vi "BBB Blink.vi"() -> ()   [LabVIEW 2025]
doc: "Automatically blink and LED attached to a digital output channel of a LINX device."
uses:
  <vilib>/MakerHub/LINX/Public/Peripherals/Digital/Digital Write N Chans.vi
  <vilib>/MakerHub/LINX/Public/Peripherals/Digital/Digital Read N Chans.vi
  <vilib>/MakerHub/LINX/Private/Local IO/LinxDigitalWrite.vi
  <vilib>/MakerHub/LINX/Public/Utilities/Check Channel.vi
  <vilib>/MakerHub/LINX/Private/Local IO/LinxDigitalRead.vi
  <vilib>/MakerHub/LINX/Private/Local IO/Handle Errors.vi
  <vilib>/MakerHub/LINX/Private/Utilties/Generate Error.vi
  <vilib>/MakerHub/LINX/Public/Peripherals/PWM/PWM Set Duty Cycle N Chans.vi
  <vilib>/MakerHub/LINX/Public/Peripherals/Digital/Digital Write 1 Chan.vi
  <vilib>/MakerHub/LINX/Public/Peripherals/Digital/Digital Read 1 Chan.vi
  <vilib>/MakerHub/LINX/Public/Utilities/Open Local.vi
  <vilib>/MakerHub/LINX/LMH-LINX.lvlib
panel:
  out "DI Value":bool
  in  "Digital Input Channel":u8=8
  out "DO Value":bool
  in  "Digital Output Channel":u8=7
  out "Loop Rate (Hz)":u32=4
  in  "Stop Button":bool
  # "LINX Device Settings"
  # "LED Value"
  # "Blink (Serial Interface)\n\nThis example demonstrates how to blink an LED on a LINX device connected to \nthe host computer using USB / Serial.\n\nInstructions\n1. Select the Serial Port associated with the LINX Device.\n2. Select the Digital Pin connected to the LED.\n3. Click the Run Arrow."
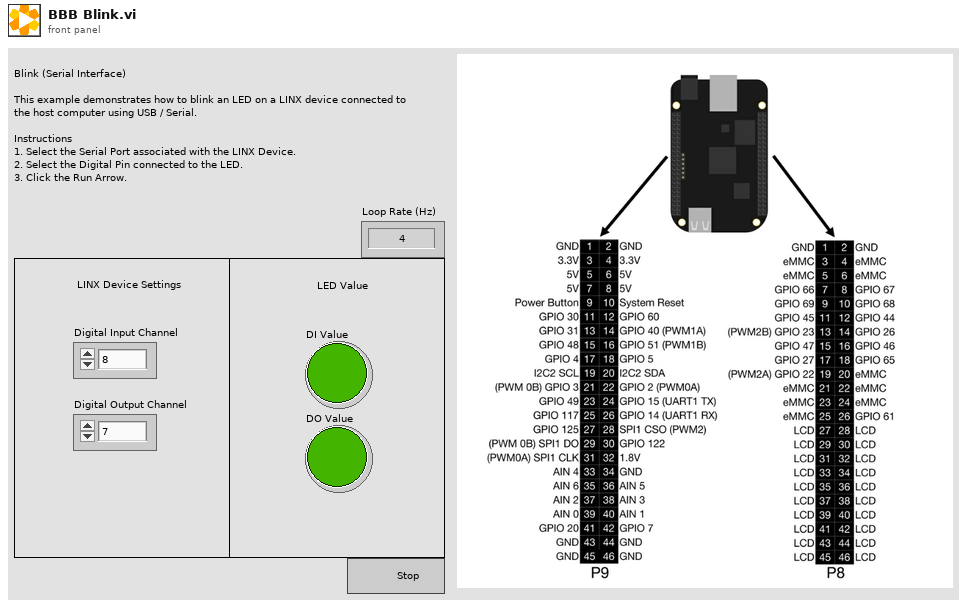
[diagram p1: front panel]
types:
  T1 = typedef "LMH-LINX.lvlib/LINX Ref.ctl" = cluster{"IO":T2, "Interface":T3, "LINX Device Config":T4}
  T2 = typedef "LMH-LINX.lvlib/Platform.ctl" = enum16{"Remote", "Local"}
  T3 = typedef "LMH-LINX.lvlib/Interface.ctl" = enum16{"Serial", "TCP"}
  T4 = typedef "LMH-LINX.lvlib/Device.lvlib/LINX Device Config.ctl" = cluster{"Interface":T3, "COM Port":refnum<visa-resource-name>, "TCP Configuration":T5, "Device Family":u8, "Device ID":u8, "Device Name":string, "TCP Ref":refnum<k5>, "Channels":T6}
  T5 = typedef "LMH-LINX.lvlib/Device.lvlib/TCP Config.ctl" = cluster{"IP Address":string, "Port":u16}
  T6 = typedef "LMH-LINX.lvlib/Channels.ctl" = cluster{"DI":u8[], "DO":u8[], "AI":u8[], "AO":u8[], "PWM":u8[], "QE":u8[], "UART":u8[], "I2C 2":u8[], "SPI":u8[], "CAN":u8[], "Servo":u8[], "AI Ref (V)":dbl, "AI Resolution (Bits)":u8, "AO Ref (V)":dbl, "AO Resolution (Bits)":u8}
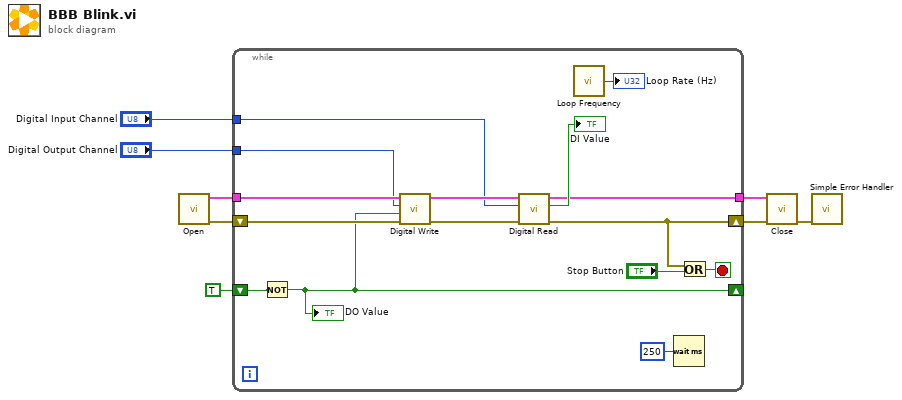
[diagram p0: block diagram]
diagram:
  n1 = call-poly <vilib>:"Open.vi"() -> ("Error Out"=w7:errorcluster, "LINX Resource"=w8:T1)  [unwired: 9 in, 1 out]
  n2 = while {
    tunnel: w8 -> [w20]
    tunnel: [w9] -> w6
    shift-right: [w10] -> w5
    shift-left: w7 -> [w19]
    shift-right: [w15] -> _
    shift-left: TRUE -> [w16]
    tunnel: "Digital Output Channel" -> [w17]
    tunnel: "Digital Input Channel" -> [w12]
    stop <- w23 stop-if-true
    n3 = Not(x=w16) -> (.not. x?=w15:bool)
    "DO Value" <- w15
    n4 = call-poly <vilib>:"Digital Write.vi"("Error In"=w19, "Output Value"=w15, "DO Channel"=w17, "LINX Resource"=w20) -> ("Error Out"=w14:errorcluster, "LINX Resource"=w13:T1)  [unwired: 6 in]
    n5 = call-poly <vilib>:"Digital Read.vi"("Error In"=w14, "DI Channel"=w12, "LINX Resource"=w13) -> ("Error Out"=w10:errorcluster, "DI Value"=→"DI Value":bool, "LINX Resource"=w9:T1)  [unwired: 6 in]
    n6 = call <vilib>:"Loop Frequency.vi"() -> ("Loop Rate (Hz)"=→"Loop Rate (Hz)":u32)
    n7 = Wait (ms)(milliseconds to wait=u32 250) -> ()  [unwired: 1 out]
    n8 = Or(x=w10, y="Stop Button") -> (x .or. y?=w23:bool)
  }
  n9 = call <vilib>:"Close.vi"("Error In"=w5, "LINX Resource"=w6) -> ("Error Out"=w4:errorcluster)  [unwired: 9 in]
  n10 = call <vilib>:"Simple Error Handler.vi"("error in (no error)"=w4) -> ()  [unwired: 4 in, 5 out]
